vi "sync and trig.vi"(8 "error in (no error)":errorcluster, 10 "time calibrate":dbl[](array[numeric]), 11 "5785_2_X_400MHz_Rx_as_scop in":refnum<class "5785_2_X_400MHz_Rx_as_scop.lvclass">) -> (0 "error out":errorcluster, 3 "5785_2_X_400MHz_Rx_as_scop out":refnum<class "5785_2_X_400MHz_Rx_as_scop.lvclass">)   [LabVIEW 2021, in "5785_2_X_400MHz_Rx_as_scop.lvclass"]
uses:
  5785_2_X_400MHz_Rx_as_scop.lvclass
  5785_2_X_400MHz_Rx_as_scop.lvclass/5785_2_X_400MHz_Rx_as_scop.ctl
  <vilib>/Utility/error.llb/Error Cluster From Error Code.vi
  <vilib>/rvi/errors/niLvFpgaAdjustHostInterfaceError.vi
  <instrlib>/_niInstr/Streaming/v1/Host/Public/Start Continuous Stream.vi
  <vilib>/rvi/interface/nirviReadWriteControl/nirviReadWriteControl.xnode
  <resource>/objmgr/sessionReference.rc
  NiFpgaLv.dll
  <vilib>/rvi/interface/Simulation/niFpgaSimulationCallBeginRW.vi
  <instrlib>/_niInstr/Streaming/v1/Host/niInstr Streaming v1 Host.lvlib
  <instrlib>/FlexRIO/API/Host/v1/NI FlexRIO API v1.lvlib
  <resource>/objmgr/niflexrioapi.rc
  <instrlib>/FlexRIO/API/Host/v1/NI FlexRIO/API/Get Property Reference - Fpga Small.vi
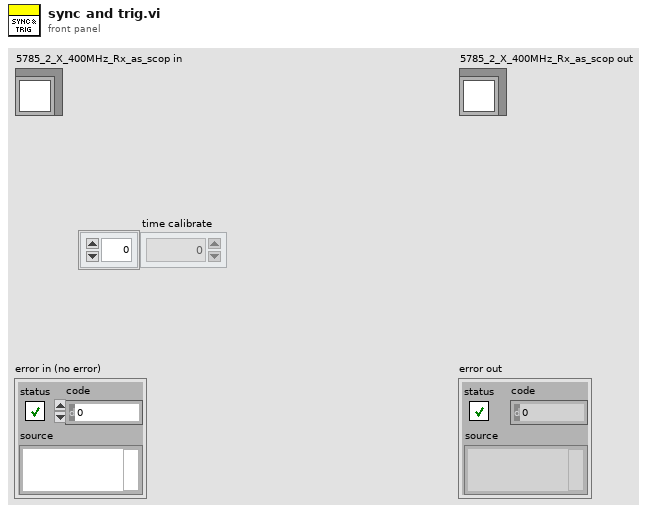
[diagram p1: front panel]
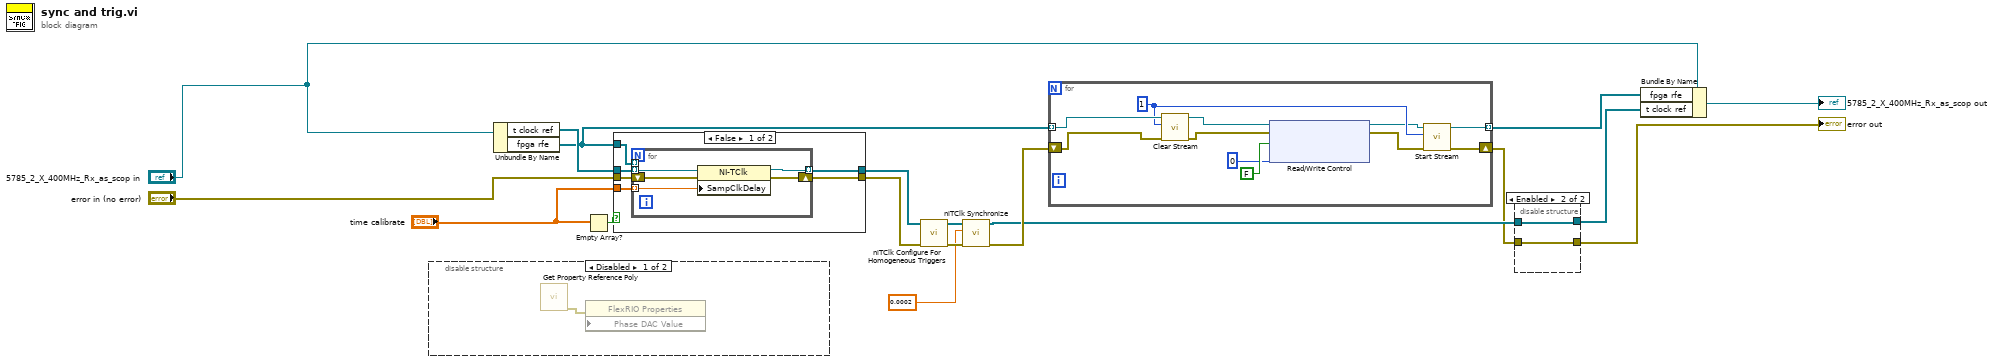
[diagram p0: block diagram]
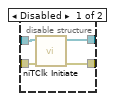
[diagram p2: hidden frame]
diagram:
  n1 = disable-structure shown="Disabled" {
    frame Disabled {
      n2 = call-poly <instrlib>:"Get Property Reference Poly.vi"() -> ("error out"=w19:errorcluster)  [unwired: 6 in, 2 out]
      n3 = property class="FlexRIO Properties" props=["Phase DAC Value"](error in=w19) -> ()  [unwired: 2 in, 2 out]
    }
    frame Enabled {
    }
  }
  n4 = Unbundle By Name("5785_2_X_400MHz_Rx_as_scop in") -> ("t clock ref"=w11:refnum<k20>[], "fpga rfe"=w1:refnum<k20>[])
  n5 = Empty Array?(array="time calibrate") -> (empty?=w7:bool)
  n6 = case shown="False" w7 {
    tunnel: "error in (no error)" -> [w25 w32]
    tunnel: [w24 w32] -> w12
    tunnel: w11 -> [w23 w31]
    tunnel: [w22 w31] -> w10
    tunnel: "time calibrate" -> [w21 _]
    tunnel: w1 -> [w20 _]
    frame False {
      n7 = for {
        tunnel: w23 -> [w30] mode=indexing
        tunnel: [w29] -> w22 mode=indexing
        shift-right: [w28] -> w24
        shift-left: w25 -> [w27]
        tunnel: w21 -> [w26] mode=indexing
        tunnel: w20 -> [_] mode=indexing
        n8 = property class="NI-TClk"(reference=w30, error in=w27, "SampClkDelay"=w26) -> (reference out=w29:refnum<k20>, error out=w28:errorcluster)
      }
    }
    frame True {
    }
  }
  n9 = call <instrlib>:"niTClk Configure For Homogeneous Triggers.vi"("error in (no error)"=w12, "sessions"=w10) -> ("error out"=w16:errorcluster, "sessions out"=w17:refnum<k20>[])  [unwired: 8 in]
  n10 = call <instrlib>:"niTClk Synchronize.vi"("error in (no error)"=w16, "minimum T clock period"=0.0002, "sessions"=w17) -> ("error out"=w18:errorcluster, "sessions out"=w6:refnum<k20>[])  [unwired: 7 in]
  n11 = for {
    tunnel: w1 -> [w41] mode=indexing
    shift-right: [w33] -> w5
    shift-left: w18 -> [w39]
    tunnel: [w34] -> w9 mode=indexing
    w37 = 1 ("stream index")
    n12 = call <instrlib>:"Clear Stream.vi"("error in (no error)"=w39, "stream index"=w37, "refnum in"=w41) -> ("error out"=w38:errorcluster, "refnum out"=w40:refnum<k20>)  [unwired: 7 in]
    n13 = xnode "Read/Write Control"("FPGA VI Reference In"=w40, "error in"=w38, "reset system clock"=FALSE, "rx count .5"=u32 0 ("num of points to send")) -> ("FPGA VI Reference Out"=w35:refnum<k20>, "error out"=w36:errorcluster)
    n14 = call-poly <instrlib>:"Start Stream.vi"("error in (no error)"=w36, "stream index"=w37, "refnum in"=w35) -> ("error out"=w33:errorcluster, "refnum out"=w34:refnum<k20>)  [unwired: 7 in]
  }
  n15 = disable-structure shown="Enabled" {
    disable-tunnel: w6 -> [w47 w49]
    disable-tunnel: w5 -> [w46 w48]
    disable-tunnel: [w45 w49] -> w4
    disable-tunnel: [w44 w48] -> w3
    frame Disabled {
      n16 = call <instrlib>:"niTClk Initiate.vi"("error in (no error)"=w46, "sessions"=w47) -> ("error out"=w44:errorcluster, "sessions out"=w45:refnum<k20>[])  [unwired: 8 in]
    }
    frame Enabled {
    }
  }
  "error out" <- w3
  n17 = Bundle By Name(cluster="5785_2_X_400MHz_Rx_as_scop in", "fpga rfe"=w9, "t clock ref"=w4) -> (→"5785_2_X_400MHz_Rx_as_scop out":refnum<class "5785_2_X_400MHz_Rx_as_scop.lvclass">)
